vi "OP600ZP_PreCharge.vi"(10 "PR":string, 11 "Tableau en entrée":string[][](array[string])) -> (3 "Tableau en sortie":string[][](array[string]), 4 "PASS?":bool[](array[boolean]))   [LabVIEW 2020]
uses:
  VG/OCV.vi
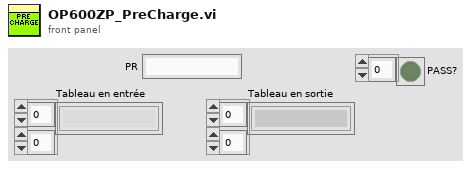
[diagram p1: front panel]
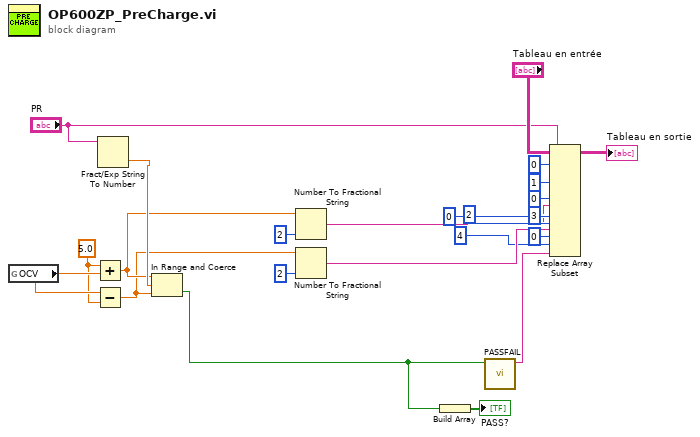
[diagram p0: block diagram]
diagram:
  w6 = 5.0 ("x")
  n1 = global read "OCV.vi" "OCV"() -> (w7:dbl)
  n2 = Add(x=w6, y=w7) -> (x+y=w2:dbl)
  n3 = Subtract(x=w7, y=w6) -> (x-y=w1:dbl)
  n4 = Fract/Exp String To Number(string="PR") -> (number=w5:dbl)  [unwired: 3 in, 1 out]
  n5 = In Range and Coerce(upper limit=w2, x=w5, lower limit=w1) -> (In Range?=w4:bool)  [unwired: 1 out]
  n6 = Number To Fractional String(number=w2, precision (6)=i16 2 ("précision (6)")) -> (F-format string=w18:string)  [unwired: 2 in]
  n7 = Number To Fractional String(number=w1, precision (6)=i16 2 ("précision (6)")) -> (F-format string=w21:string)  [unwired: 2 in]
  n8 = Build Array(w4) -> (→"PASS?":bool[])
  n9 = call <vilib>:"PASSFAIL.vi"("E"=w4) -> ("S"=w9:string)  [unwired: 10 in]
  n10 = Replace Array Subset(array="Tableau en entrée", new element #1="PR", index (row) #1=0 ("indice (ligne)"), index (col) #1=1 ("indice désactivé (col)"), new element #2=w18, index (row) #2=0 ("indice (ligne)"), index (col) #2=3 ("indice désactivé (col)"), new element #3=w21, index (row) #3=0 ("indice (ligne)"), index (col) #3=2 ("indice désactivé (col)"), new element #4=w9, index (row) #4=0 ("indice désactivé (ligne)"), index (col) #4=4 ("indice désactivé (col)")) -> (→"Tableau en sortie":string[][])
